vi "reactor_merge.vi"(10 "reactor_path":path) -> ()   [LabVIEW 2019]
uses:
  lib/libSimulationControl/libSimulationControl.lvlib
  lib/libFileFunctions/libFileFunctions.lvlib
panel:
  # "*******************************************************************\nBiogas Plant Control\n\nAuthor: Paul Zügel\nGCSC-Frankfurt am Main 2020\n\n*******************************************************************"
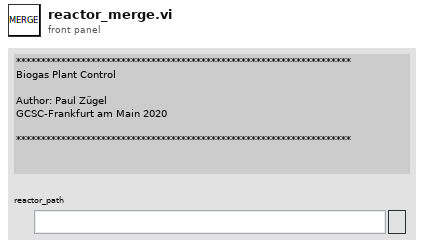
[diagram p1: front panel]
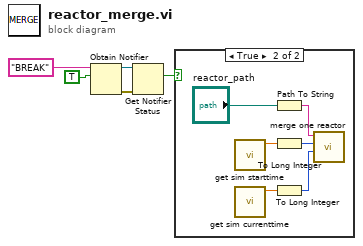
[diagram p0: block diagram]
diagram:
  n1 = Obtain Notifier(name (unnamed)="BREAK", notification data type=TRUE) -> (notifier out=w3:refnum<notifier>, error out=w2:errorcluster)  [unwired: 2 in, 1 out]
  n2 = Get Notifier Status(notifier=w3, error in (no error)=w2) -> (current notification=w1:bool)  [unwired: 4 out]
  n3 = case shown="True" w1 {
    frame False {
    }
    frame True {
      n4 = call "get sim starttime.vi"() -> ("sim_starttime"=w9:dbl)  [unwired: 10 in, 1 out]
      n5 = call "get sim currenttime.vi"() -> ("current_time"=w10:dbl)  [unwired: 10 in, 1 out]
      n6 = Path To String(path="reactor_path") -> (string=w8:string)
      n7 = To Long Integer(number=w9) -> (32bit integer=w7:i32)
      n8 = To Long Integer(number=w10) -> (32bit integer=w6:i32)
      n9 = call "merge one reactor.vi"("current_starttime"=w6, "simulation_starttime"=w7, "working_dir"=w8) -> ()  [unwired: 8 in, 1 out]
    }
  }
